vi "Create Spectrum.vi"(8 "error in (no error)":errorcluster, 11 "waveform in":waveform(dbl)) -> (0 "error out":errorcluster, 3 "Cluster":cluster{"Ramp Pattern":dbl[], "magnitude":dbl[]})   [LabVIEW 2024]
uses:
  <vilib>/measure/maspectr.llb/Power Spectrum and PSD Export Mode.ctl
  <vilib>/Analysis/4window.llb/windowTd.ctl
  <vilib>/Analysis/1siggen.llb/Ramp Pattern by Samples.vi
  <vilib>/measure/maspectr.llb/FFT Power Spectrum and PSD for 1 Chan.vi
  <vilib>/measure/NI_MAPro.lvlib
  <vilib>/Analysis/NI_AALBase.lvlib
  <vilib>/Analysis/NI_AALPro.lvlib
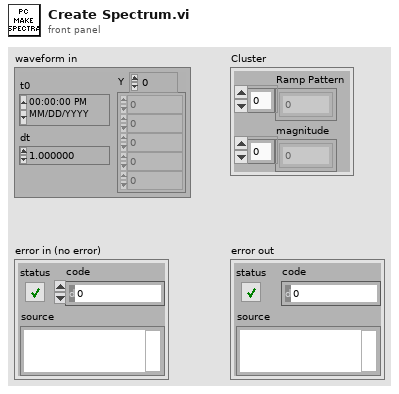
[diagram p1: front panel]
types:
  T1 = typedef "NI_AALPro.lvlib/windowTd.ctl" = u32
  T2 = cluster{"averaging mode":enum16{"No averaging", "Vector averaging", "RMS averaging", "Peak hold"}, "weighting mode":enum16{"Linear", "Exponential"}, "number of averages":u32}
  T3 = typedef "NI_MAPro.lvlib/Power Spectrum and PSD Export Mode.ctl" = u16
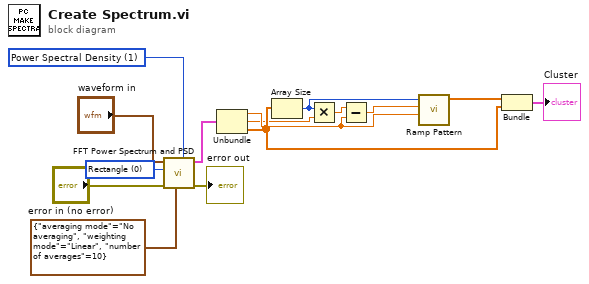
[diagram p0: block diagram]
diagram:
  w1 = T1 0 items=["Rectangle"=0, "Hanning"=1, "Hamming"=2, "Blackman-Harris"=3, "Exact Blackman"=4, "Blackman"=5, "Flat Top"=6, "4 Term B-Harris "=7, "7 Term B-Harris"=8, "Low Sidelobe"=9, "Blackman Nuttall"=11, "Triangle"=30, "Bartlett-Hanning"=31, "Bohman"=32, "Parzen"=33, "Welch"=34, "Kaiser"=60, "Dolph-Chebyshev"=61, "Gaussian"=62] ("window")
  w4 = T3 1 items=["Power Spectrum", "Power Spectral Density"] ("export mode")
  n1 = call-poly <vilib>:"FFT Power Spectrum and PSD.vi"("export mode"=w4, "averaging parameters"=T2 {"averaging mode"=enum."No averaging", "weighting mode"=enum."Linear", "number of averages"=10}, "error in (no error)"="error in (no error)", "window"=w1, "time signal"="waveform in") -> ("error out"=→"error out":errorcluster, "Power Spectrum / PSD"=w6:cluster{"f0":dbl, "df":dbl, "magnitude":dbl[]})  [unwired: 3 in, 2 out]
  n2 = Unbundle(w6) -> ("f0"=w9:dbl, "df"=w7:dbl, "magnitude"=w13:dbl[])
  n3 = Array Size(array=w13) -> (size(s)=w8:i32)
  n4 = Multiply(x=w8, y=w7) -> (x*y=w10:dbl)
  n5 = Subtract(x=w10, y=w9) -> (x-y=w11:dbl)
  n6 = call-poly <vilib>:"Ramp Pattern.vi"("start"=w9, "end"=w11, "samples"=w8) -> ("Ramp Pattern"=w12:dbl[])  [unwired: 7 in, 1 out]
  n7 = Bundle("Ramp Pattern"=w12, "magnitude"=w13) -> (→"Cluster":cluster{"Ramp Pattern":dbl[], "magnitude":dbl[]})  [unwired: 1 in]
